vi "MLin-构造矩形区域1.vi"(8 "转角":dbl, 9 "高":sgl, 10 "宽":sgl, 11 "中心点":cluster{"X":sgl, "Y":sgl}={"X"=0.5, "Y"=0.5}) -> (3 "斜矩形":T1 {"Rotation" format="%.2f"; "Left" scale=0.0..1024.0; "Right" scale=0.0..1024.0})   [LabVIEW 2018]
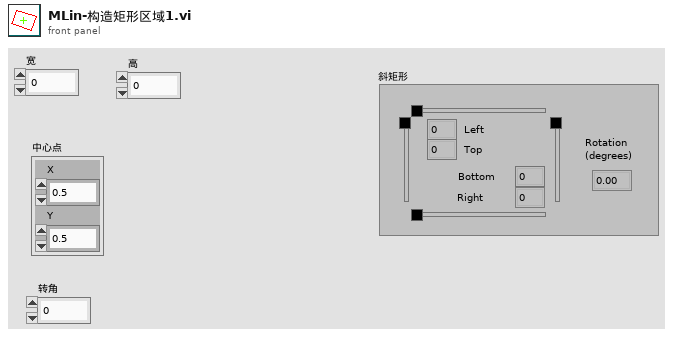
[diagram p1: front panel]
types:
  T1 = typedef "IMAQ Rectangle" = cluster{"Left":i32, "Top":i32, "Right":i32, "Bottom":i32, "Rotation":dbl}
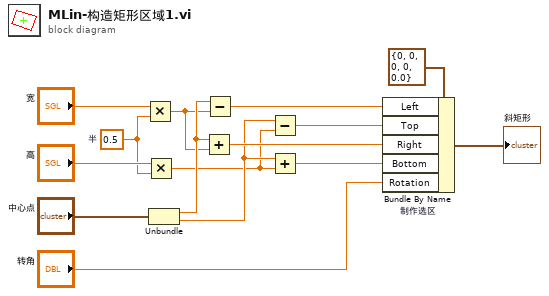
[diagram p0: block diagram]
diagram:
  w5 = sgl 0.5  # 半
  n1 = Multiply(x="宽", y=w5) -> (x*y=w4:sgl)
  n2 = Multiply(x="高", y=w5) -> (x*y=w3:sgl)
  n3 = Unbundle("中心点") -> ("X"=w10:sgl, "Y"=w9:sgl)
  n4 = Add(x=w10, y=w4) -> (x+y=w14:sgl)
  n5 = Subtract(x=w10, y=w4) -> (x-y=w12:sgl)
  n6 = Subtract(x=w9, y=w3) -> (x-y=w13:sgl)
  n7 = Add(x=w9, y=w3) -> (x+y=w15:sgl)
  n8 = Bundle By Name "制作选区"(cluster=T1 {"Left"=0, "Top"=0, "Right"=0, "Bottom"=0, "Rotation"=0.0} ("Rectangle"), "Left"=w12, "Top"=w13, "Right"=w14, "Bottom"=w15, "Rotation"="转角") -> (→"斜矩形":T1)
